vi "MecaWheel_normalize.vi"(9 "MaxAttainableSpeed":dbl format="%19.3f", 11 "in MECA_WHEEL_SPEEDS":T1 {"RearRightSpeed" format="%19.3f"; "RearLeftSpeed" format="%19.3f"; "FrontRightSpeed" format="%19.3f"; "FrontLeftSpeed" format="%19.3f"}) -> (3 "out MECA_WHEEL_SPEEDS":T1 {"RearRightSpeed" format="%19.3f"; "RearLeftSpeed" format="%19.3f"; "FrontRightSpeed" format="%19.3f"; "FrontLeftSpeed" format="%19.3f"})   [LabVIEW 2019, in "Trajectory_Library.lvlib"]
doc: "Normalizes the wheel speeds using some max attainable speed. Sometimes, after inverse kinematics, the requested speed from a/several modules may be above the max attainable speed for the driving motor on that module. To fix this issue, one can \"normalize\" all the wheel speeds to make sure that all requested module speeds are below the absolute threshold, while maintaining the ratio of speeds between modules.\n\nParameters:\n - in Meca_wheel_speeds - Data structure\n - MaxAttainableSpeed - The absolute max speed that a wheel can reach.\n\nReturns:\n - out Meca_wheel_speeds - Data structure"
uses:
  Trajectory_Library.lvlib
  MECA_WHEEL_SPEEDS.ctl
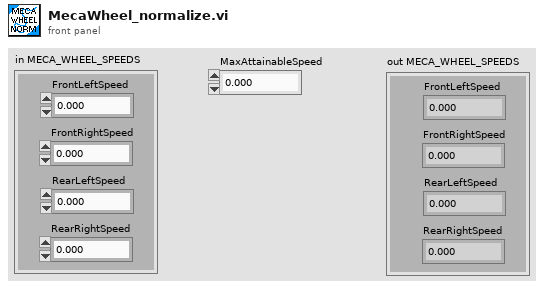
[diagram p1: front panel]
types:
  T1 = typedef "Trajectory_Library.lvlib/MECA_WHEEL_SPEEDS.ctl" = cluster{"FrontLeftSpeed":dbl, "FrontRightSpeed":dbl, "RearLeftSpeed":dbl, "RearRightSpeed":dbl}
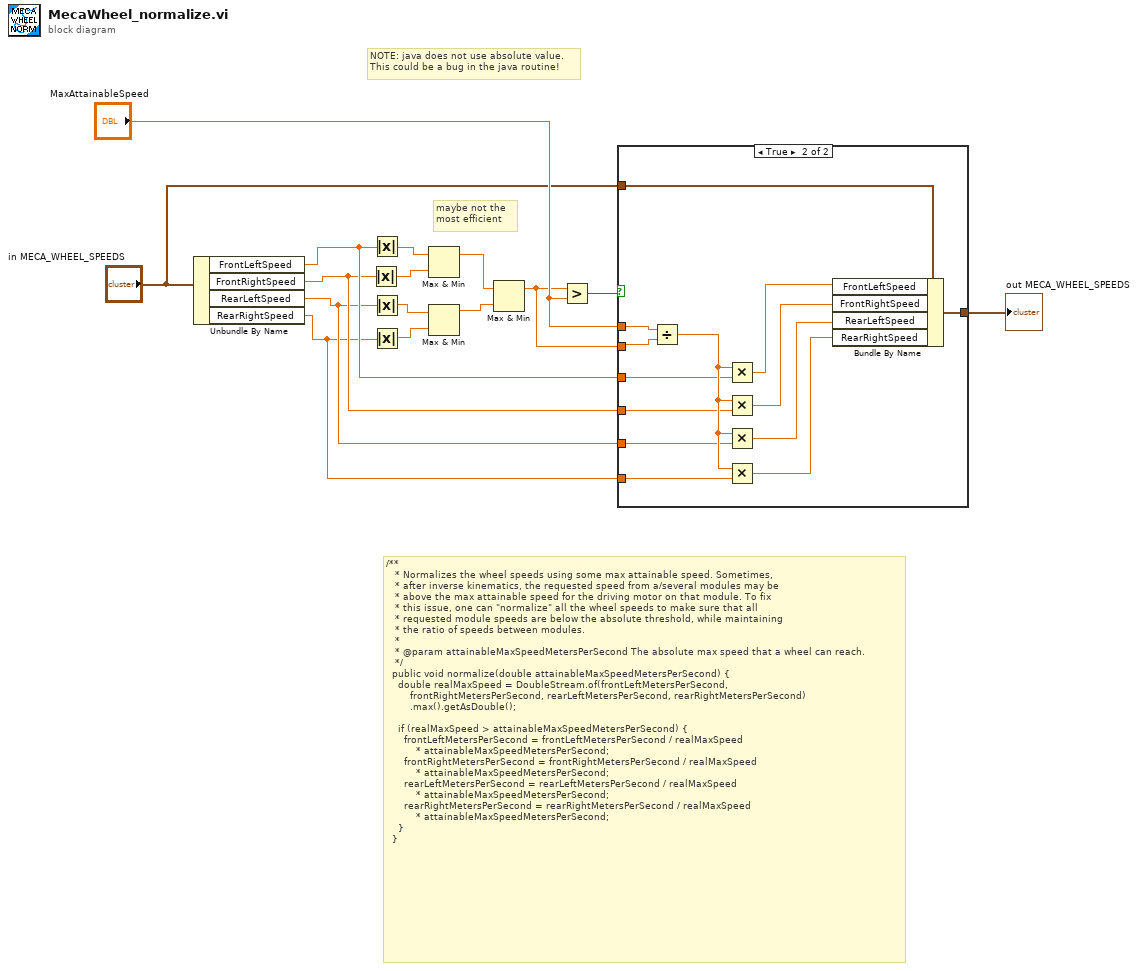
[diagram p0: block diagram]
diagram:
  # "NOTE: java does not use absolute value.\nThis could be a bug in the java routine!"
  # "maybe not the \nmost efficient"
  # "/**\n   * Normalizes the wheel speeds using some max attainable speed. Sometimes,\n   * after inverse kinematics, the requested speed from a/several modules may be\n   * above the max attainable speed for the driving motor on that module. To fix\n   * this issue, one can \"normalize\" all the wheel speeds to make sure that all\n   * requested module speeds are below the absolute threshold, while maintaining\n   * the ratio of speeds between modules.\n   *\n   * @param attainableMaxSpeedMetersPerSecond The absolute max speed that a wheel can reach.\n   */\n  public void normalize(double attainableMaxSpeedMetersPerSecond) {\n    double realMaxSpeed = DoubleStream.of(frontLeftMetersPerSecond,\n        frontRightMetersPerSecond, rearLeftMetersPerSecond, rearRightMetersPerSecond)\n        .max().getAsDouble();\n\n    if (realMaxSpeed > attainableMaxSpeedMetersPerSecond) {\n      frontLeftMetersPerSecond = frontLeftMetersPerSecond / realMaxSpeed\n          * attainableMaxSpeedMetersPerSecond;\n      frontRightMetersPerSecond = frontRightMetersPerSecond / realMaxSpeed\n          * attainableMaxSpeedMetersPerSecond;\n      rearLeftMetersPerSecond = rearLeftMetersPerSecond / realMaxSpeed\n          * attainableMaxSpeedMetersPerSecond;\n      rearRightMetersPerSecond = rearRightMetersPerSecond / realMaxSpeed\n          * attainableMaxSpeedMetersPerSecond;\n    }\n  }"
  n1 = Unbundle By Name("in MECA_WHEEL_SPEEDS") -> ("FrontLeftSpeed"=w8:dbl, "FrontRightSpeed"=w7:dbl, "RearLeftSpeed"=w6:dbl, "RearRightSpeed"=w5:dbl)
  n2 = Absolute Value(x=w7) -> (abs(x)=w14:dbl)
  n3 = Absolute Value(x=w8) -> (abs(x)=w15:dbl)
  n4 = Absolute Value(x=w6) -> (abs(x)=w13:dbl)
  n5 = Absolute Value(x=w5) -> (abs(x)=w12:dbl)
  n6 = Max & Min(x=w15, y=w14) -> (max(x,y)=w10:dbl)  [unwired: 1 out]
  n7 = Max & Min(x=w13, y=w12) -> (max(x,y)=w11:dbl)  [unwired: 1 out]
  n8 = Max & Min(x=w10, y=w11) -> (max(x,y)=w3:dbl)  [unwired: 1 out]
  n9 = Greater?(x=w3, y="MaxAttainableSpeed") -> (0:w9:bool)
  n10 = case shown="True" w9 {
    tunnel: w8 -> [_ w23]
    tunnel: w7 -> [_ w24]
    tunnel: w6 -> [_ w25]
    tunnel: w5 -> [_ w26]
    tunnel: "MaxAttainableSpeed" -> [_ w29]
    tunnel: w3 -> [_ w28]
    tunnel: "in MECA_WHEEL_SPEEDS" -> [w16 w22]
    tunnel: [w16 w17] -> w1
    frame False {
    }
    frame True {
      n11 = Divide(x=w29, y=w28) -> (x/y=w27:dbl)
      n12 = Multiply(x=w27, y=w23) -> (x*y=w21:dbl)
      n13 = Multiply(x=w27, y=w24) -> (x*y=w20:dbl)
      n14 = Multiply(x=w27, y=w25) -> (x*y=w19:dbl)
      n15 = Multiply(x=w27, y=w26) -> (x*y=w18:dbl)
      n16 = Bundle By Name(cluster=w22, "FrontLeftSpeed"=w21, "FrontRightSpeed"=w20, "RearLeftSpeed"=w19, "RearRightSpeed"=w18) -> (w17:T1)
    }
  }
  "out MECA_WHEEL_SPEEDS" <- w1
